vi "LAC Query (SubVI).vi"(5 "interval(ms)":u32=50, 7 "timeout(ms)":u32=500, 8 "error in":errorcluster, 9 "Command":string, 11 "VISA name in":refnum<visa-resource-name>) -> (0 "error out":errorcluster, 1 "read buffer":string, 3 "VISA name out":refnum<visa-resource-name>)   [LabVIEW 2014]
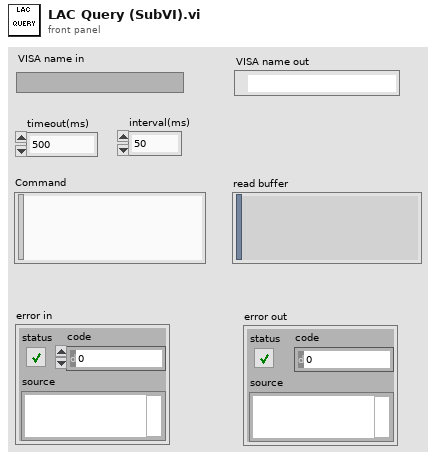
[diagram p1: front panel]
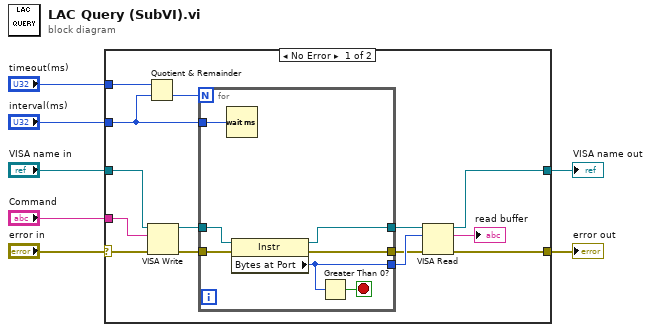
[diagram p0: block diagram]
diagram:
  n1 = case shown="No Error" "error in" {
    selector: "error in" -> [w12 w30]
    tunnel: "VISA name in" -> [w16 w29]
    tunnel: [w15 w29] -> w6
    tunnel: [w13 w30] -> w5
    tunnel: "Command" -> [w9 _]
    tunnel: "timeout(ms)" -> [w11 _]
    tunnel: "interval(ms)" -> [w8 _]
    frame No Error {
      n2 = Quotient & Remainder(x=w11, y=w8) -> (floor(x/y)=w18:u32)  [unwired: 1 out]
      n3 = VISA Write(VISA resource name=w16, write buffer=w9, error in (no error)=w12) -> (VISA resource name out=w21:refnum<visa-resource-name>, error out=w17:errorcluster)  [unwired: 1 out]
      n4 = for {
        N: w18 -> [_]
        tunnel: w21 -> [w27]
        tunnel: [w25] -> w20
        tunnel: [w26] -> w19
        tunnel: w17 -> [w24]
        tunnel: [w23] -> w14
        tunnel: w8 -> [w22]
        stop <- w28 stop-if-true
        n5 = Wait (ms)(milliseconds to wait=w22) -> ()  [unwired: 1 out]
        n6 = property class="Instr"(reference=w27, error in=w24) -> (reference out=w26:refnum<visa-resource-name>, error out=w23:errorcluster, "Bytes at Port"=w25:u32)
        n7 = Greater Than 0?(x=w25) -> (x > 0?=w28:bool)
      }
      n8 = VISA Read(VISA resource name=w19, byte count=w20, error in (no error)=w14) -> (VISA resource name out=w15:refnum<visa-resource-name>, read buffer=→"read buffer":string, error out=w13:errorcluster)  [unwired: 1 out]
    }
    frame Error {
    }
  }
  "VISA name out" <- w6
  "error out" <- w5
